vi "RS_SMBV100A_get_scenario.vi"(3 "error in":errorcluster {"code" format="%.0x"}, 5 "Scenario in":string="****************************** MOVEMENT FILE ******************************\nRESOLUTION: 50\nREFERENCE: 11.583333,48.150,500\nSTART: 0, 0, 0, 10\nSTAY: 10000\nLINE: 200, 0, 0\nLINE: 100, 0, 19.6\nLINE: 600, 0, 0\nLINE: 100, 0, -19.6\nARC: 1000, 500, 180\nLINE: -200, 0, 0\nLINE: -100, 0, 19.6\nLINE: -600, 0, 0\nLINE: -100, 0, -19.6\nARC: 0, 500, 180") -> (0 "error out":errorcluster {"code" format="%.0x"}, 2 "Scenario info":T1)   [LabVIEW 2018]
uses:
  RS_SMBV100A_ScenarioInfo.ctl
  RS_SMBV100A_ScenarioLineInfo.ctl
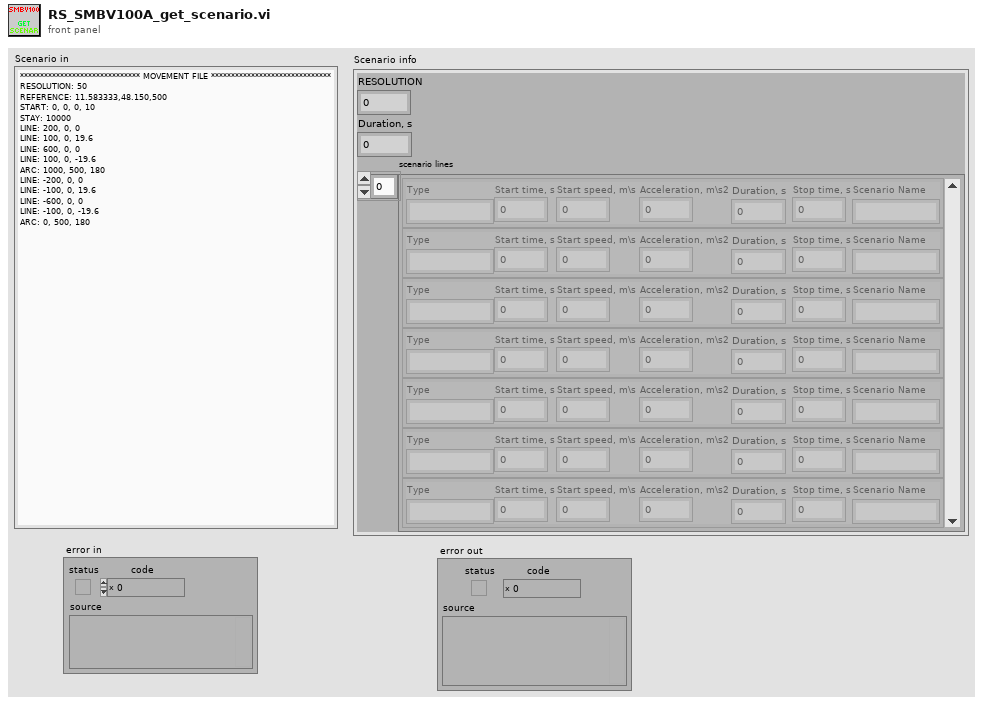
[diagram p1: front panel]
types:
  T1 = typedef "RS_SMBV100A_ScenarioInfo.ctl" = cluster{"RESOLUTION":dbl, "Duration, s":dbl, "scenario lines":T2[]}
  T2 = typedef "RS_SMBV100A_ScenarioLineInfo.ctl" = cluster{"Type":string, "Start time, s":dbl, "Start speed, m\\s":dbl, "Acceleration, m\\s2":dbl, "Duration, s":dbl, "Stop time, s":dbl, "Scenario Name":string}
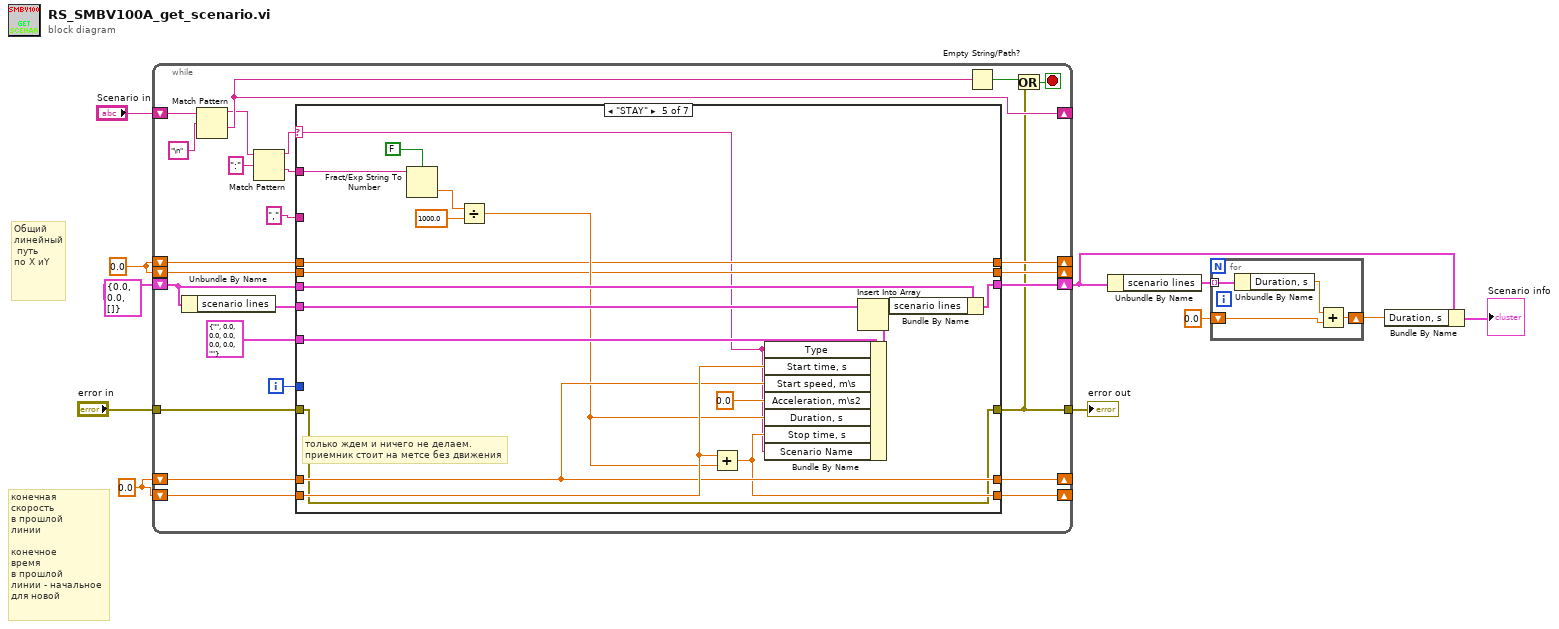
[diagram p0: block diagram]
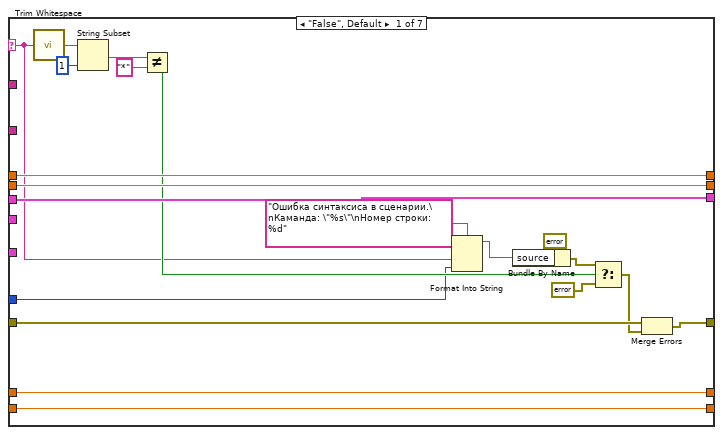
[diagram p2: hidden frame]
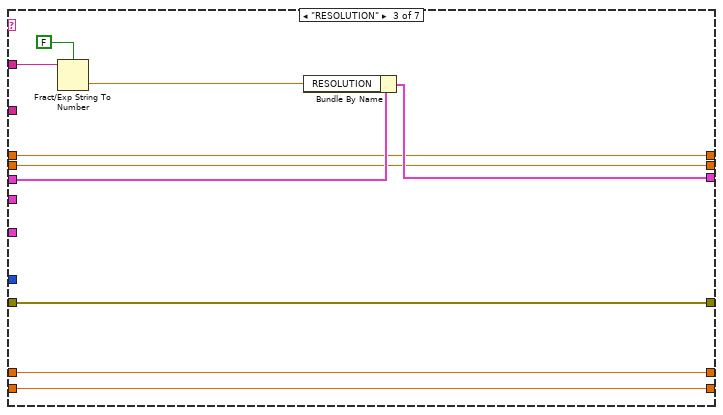
[diagram p4: hidden frame]
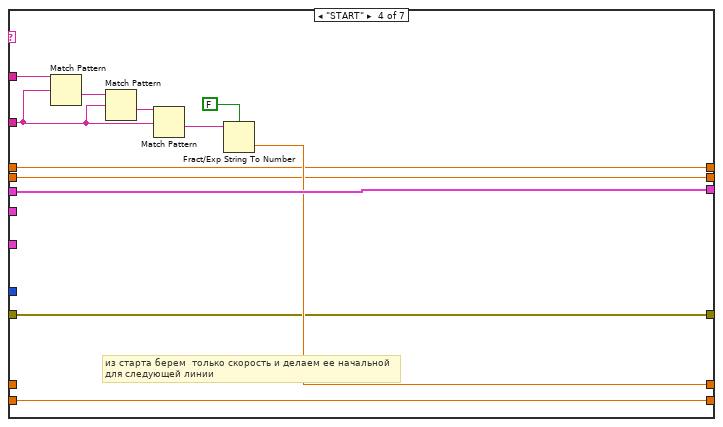
[diagram p5: hidden frame]
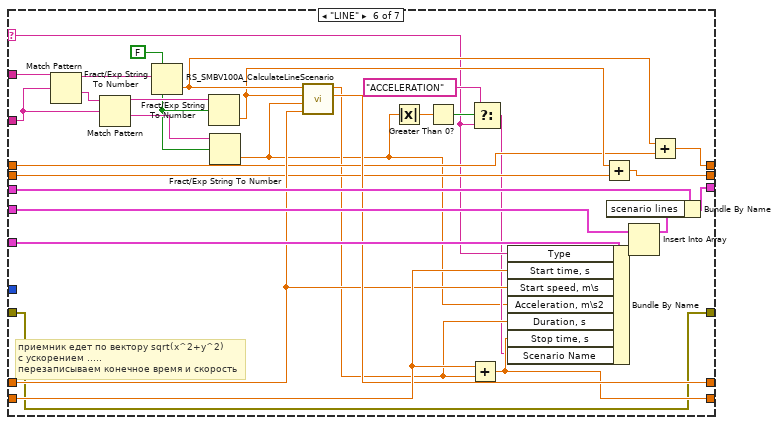
[diagram p6: hidden frame]
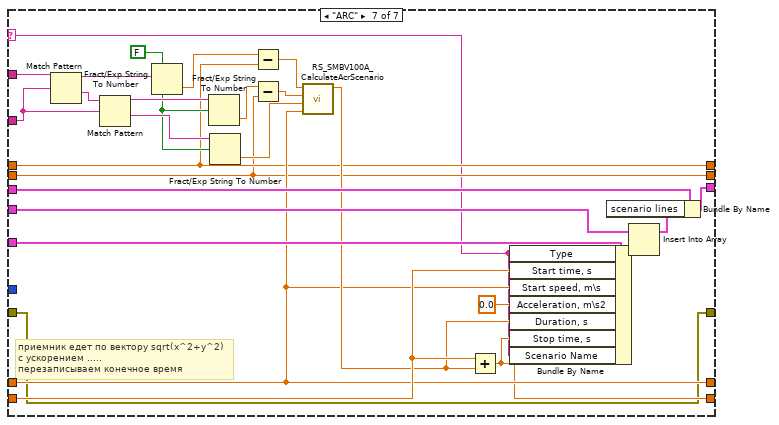
[diagram p7: hidden frame]
diagram:
  w9 = 0.0
  w10 = 0.0
  # "Общий \nлинейный\n путь \nпо X иY"
  # "конечная\nскорость\nв прошлой\nлинии\n\nконечное\nвремя\nв прошлой\nлинии - начальное \nдля новой"
  n1 = while {
    shift-right: [w34] -> _
    shift-left: "Scenario in" -> [w36]
    shift-right: [w29] -> w6
    shift-left: T1 {"RESOLUTION"=0.0, "Duration, s"=0.0, "scenario lines"=[]} ("Scenario info") -> [w23]
    shift-right: [w28] -> _
    shift-left: w10 -> [w27]
    shift-right: [w25] -> _
    shift-left: w10 -> [w26]
    shift-right: [w18] -> _
    shift-left: w9 -> [w21]
    shift-right: [w19] -> _
    shift-left: w9 -> [w20]
    tunnel: [w13] -> w2
    tunnel: "error in" -> [w14]
    i -> [w12]
    stop <- w15 stop-if-true
    n2 = Unbundle By Name(w23) -> ("scenario lines"=w22:T2[])
    n3 = Match Pattern(string=w36, regular expression="\n") -> (before substring=w33:string, after substring=w34:string)  [unwired: 1 in, 2 out]
    n4 = Match Pattern(string=w33, regular expression=":") -> (before substring=w31:string, after substring=w30:string)  [unwired: 1 in, 2 out]
    n5 = case shown="\"STAY\"" w31 {
      selector: w31 -> [w38 _ _ _ w85 w107 w135]
      tunnel: w30 -> [_ _ w72 w82 w93 w134 w161]
      tunnel: [w56 w62 w69 w83 w101 w132 w159] -> w29
      tunnel: w23 -> [w56 w62 w70 w83 w102 w133 w160]
      tunnel: [w55 w61 w67 w76 w95 w120 w144] -> w28
      tunnel: w27 -> [w55 w61 w67 _ w95 w119 w144]
      tunnel: w26 -> [w54 w60 w66 w84 w96 w127 w154]
      tunnel: [w54 w60 w66 w84 w87 w111 w137] -> w25
      tunnel: "," ("regular expression") -> [_ _ _ w79 _ w125 w152]
      tunnel: w22 -> [_ _ _ _ w99 w130 w157]
      tunnel: T2 {"Type"="", "Start time, s"=0.0, "Start speed, m\\s"=0.0, "Acceleration, m\\s2"=0.0, "Duration, s"=0.0, "Stop time, s"=0.0, "Scenario Name"=""} ("Scenario info") -> [_ _ _ _ w98 w129 w156]
      tunnel: w21 -> [w53 w59 w65 w75 w88 w114 w141]
      tunnel: w20 -> [w52 w58 w64 w74 w89 w113 w139]
      tunnel: [w52 w58 w64 w74 w89 w118 w139] -> w19
      tunnel: [w53 w59 w65 w75 w88 w116 w141] -> w18
      tunnel: [w46 w57 w63 w73 w86 w110 w136] -> w13
      tunnel: w14 -> [w47 w57 w63 w73 w86 w110 w136]
      tunnel: w12 -> [w37 _ _ _ _ _ _]
      frame "False", Default {
        n6 = call <vilib>:"Trim Whitespace.vi"("string"=w38) -> ("trimmed string"=w48:string)  [unwired: 1 in]
        n7 = String Subset(string=w48, length (rest)=1 ("length (rest)")) -> (substring=w50:string)  [unwired: 1 in]
        n8 = Not Equal?(x=w50, y="*") -> (x != y?=w45:bool)
        n9 = Format Into String(format string="Ошибка синтаксиса в сценарии.\nКаманда: \"%s\"\nНомер строки: %d", w38, w37) -> (resulting string=w40:string)  [unwired: 2 in, 1 out]
        n10 = Bundle By Name(cluster=errorcluster {"status"=TRUE, "code"=5450, "source"=""} ("t"), "source"=w40) -> (w41:errorcluster)
        n11 = Select(t=w41, s=w45, f=errorcluster {"status"=FALSE, "code"=0, "source"=""} ("error in")) -> (s? t:f=w43:errorcluster)
        n12 = Merge Errors(w47, w43) -> (w46:errorcluster)
      }
      frame "REFERENCE" {
      }
      frame "RESOLUTION" {
        n13 = Fract/Exp String To Number(use system decimal point (T)=FALSE, string=w72) -> (number=w68:dbl)  [unwired: 2 in, 1 out]
        n14 = Bundle By Name(cluster=w70, "RESOLUTION"=w68) -> (w69:T1)
      }
      frame "START" {
        # "из старта берем  только скорость и делаем ее начальной\nдля следующей линии"
        n15 = Match Pattern(string=w82, regular expression=w79) -> (after substring=w81:string)  [unwired: 1 in, 3 out]
        n16 = Match Pattern(string=w81, regular expression=w79) -> (after substring=w80:string)  [unwired: 1 in, 3 out]
        n17 = Match Pattern(string=w80, regular expression=w79) -> (after substring=w77:string)  [unwired: 1 in, 3 out]
        n18 = Fract/Exp String To Number(use system decimal point (T)=FALSE, string=w77) -> (number=w76:dbl)  [unwired: 2 in, 1 out]
      }
      frame "STAY" {
        # "только ждем и ничего не делаем. \nприемник стоит на метсе без движения"
        n19 = Fract/Exp String To Number(use system decimal point (T)=FALSE, string=w93) -> (number=w91:dbl)  [unwired: 2 in, 1 out]
        n20 = Divide(x=w91, y=1000.0) -> (x/y=w90:dbl)
        n21 = Add(x=w96, y=w90) -> (x+y=w87:dbl)
        n22 = Bundle By Name(cluster=w98, "Type"=w85, "Start time, s"=w96, "Start speed, m\\s"=w95, "Acceleration, m\\s2"=0.0 ("Acceleration, m\\s2"), "Duration, s"=w90, "Stop time, s"=w87, "Scenario Name"=w85) -> (w97:T2)
        n23 = Insert Into Array(array=w99, new element=w97) -> (w100:T2[])  [unwired: 1 in]
        n24 = Bundle By Name(cluster=w102, "scenario lines"=w100) -> (w101:T1)
      }
      frame "LINE" {
        w121 = FALSE ("use system decimal point (T)")
        # "приемник едет по вектору sqrt(x^2+y^2)\nc ускорением .....\nперезаписываем конечное время и скорость"
        n25 = Match Pattern(string=w134, regular expression=w125) -> (before substring=w124:string, after substring=w126:string)  [unwired: 1 in, 2 out]
        n26 = Match Pattern(string=w126, regular expression=w125) -> (before substring=w123:string, after substring=w122:string)  [unwired: 1 in, 2 out]
        n27 = Fract/Exp String To Number(use system decimal point (T)=w121, string=w124) -> (number=w117:dbl)  [unwired: 2 in, 1 out]
        n28 = Fract/Exp String To Number(use system decimal point (T)=w121, string=w123) -> (number=w115:dbl)  [unwired: 2 in, 1 out]
        n29 = Fract/Exp String To Number(use system decimal point (T)=w121, string=w122) -> (number=w105:dbl)  [unwired: 2 in, 1 out]
        n30 = call "RS_SMBV100A_CalculateLineScenario.vi"("Start speed"=w119, "acceleration"=w105, "delta y"=w115, "delta X"=w117) -> ("Finished Speed"=w120:dbl, "Duration"=w112:dbl)  [unwired: 6 in]
        n31 = Absolute Value(x=w105) -> (abs(x)=w104:dbl)
        n32 = Greater Than 0?(x=w104) -> (x > 0?=w109:bool)
        n33 = Add(x=w127, y=w112) -> (x+y=w111:dbl)
        n34 = Select(t="ACCELERATION", s=w109, f=w107) -> (s? t:f=w106:string)
        n35 = Bundle By Name(cluster=w129, "Type"=w107, "Start time, s"=w127, "Start speed, m\\s"=w119, "Acceleration, m\\s2"=w105, "Duration, s"=w112, "Stop time, s"=w111, "Scenario Name"=w106) -> (w128:T2)
        n36 = Add(x=w115, y=w113) -> (x+y=w118:dbl)
        n37 = Insert Into Array(array=w130, new element=w128) -> (w131:T2[])  [unwired: 1 in]
        n38 = Bundle By Name(cluster=w133, "scenario lines"=w131) -> (w132:T1)
        n39 = Add(x=w117, y=w114) -> (x+y=w116:dbl)
      }
      frame "ARC" {
        w148 = FALSE ("use system decimal point (T)")
        # "приемник едет по вектору sqrt(x^2+y^2)\nc ускорением .....\nперезаписываем конечное время"
        n40 = Match Pattern(string=w161, regular expression=w152) -> (before substring=w151:string, after substring=w153:string)  [unwired: 1 in, 2 out]
        n41 = Match Pattern(string=w153, regular expression=w152) -> (before substring=w150:string, after substring=w149:string)  [unwired: 1 in, 2 out]
        n42 = Fract/Exp String To Number(use system decimal point (T)=w148, string=w151) -> (number=w143:dbl)  [unwired: 2 in, 1 out]
        n43 = Fract/Exp String To Number(use system decimal point (T)=w148, string=w150) -> (number=w140:dbl)  [unwired: 2 in, 1 out]
        n44 = Fract/Exp String To Number(use system decimal point (T)=w148, string=w149) -> (number=w146:dbl)  [unwired: 2 in, 1 out]
        n45 = Subtract(x=w143, y=w141) -> (x-y=w142:dbl)
        n46 = Subtract(x=w140, y=w139) -> (x-y=w138:dbl)
        n47 = call "RS_SMBV100A_CalculateAcrScenario.vi"("Start speed"=w144, "Z"=w146, "Y"=w138, "X"=w142) -> ("Duration"=w147:dbl)  [unwired: 7 in]
        n48 = Add(x=w154, y=w147) -> (x+y=w137:dbl)
        n49 = Bundle By Name(cluster=w156, "Type"=w135, "Start time, s"=w154, "Start speed, m\\s"=w144, "Acceleration, m\\s2"=0.0 ("Acceleration, m\\s2"), "Duration, s"=w147, "Stop time, s"=w137, "Scenario Name"=w135) -> (w155:T2)
        n50 = Insert Into Array(array=w157, new element=w155) -> (w158:T2[])  [unwired: 1 in]
        n51 = Bundle By Name(cluster=w160, "scenario lines"=w158) -> (w159:T1)
      }
    }
    n52 = Empty String/Path?(string/path=w34) -> (empty?=w16:bool)
    n53 = Or(x=w16, y=w13) -> (x .or. y?=w15:bool)
  }
  "error out" <- w2
  n54 = Unbundle By Name(w6) -> ("scenario lines"=w8:T2[])
  n55 = for {
    tunnel: w8 -> [w165] mode=indexing
    shift-right: [w164] -> w5
    shift-left: 0.0 ("Duration, s") -> [w162]
    n56 = Unbundle By Name(w165) -> ("Duration, s"=w163:dbl)
    n57 = Add(x=w163, y=w162) -> (x+y=w164:dbl)
  }
  n58 = Bundle By Name(cluster=w6, "Duration, s"=w5) -> (→"Scenario info":T1)
